vi "Find_Unmoving_Dots_in_(X,Y)-6.vi"(4 "error IN":errorcluster, 5 "Gaps for closing":i32, 6 "dR min":dbl, 7 "[IN] Primary (X,Y)":dbl[][](array[numeric])) -> (0 "error OUT":errorcluster, 1 "[OUT] Stationary Dots":T1(array[cluster]), 2 "[OUT] Dot matrix\nwith statuses for\nmoving and poten-\ntially moving dots":i16[][](array[numeric]), 3 "[OUT] (X,Y) Potentially Moving":dbl[][](array[numeric]))   [LabVIEW 2013]
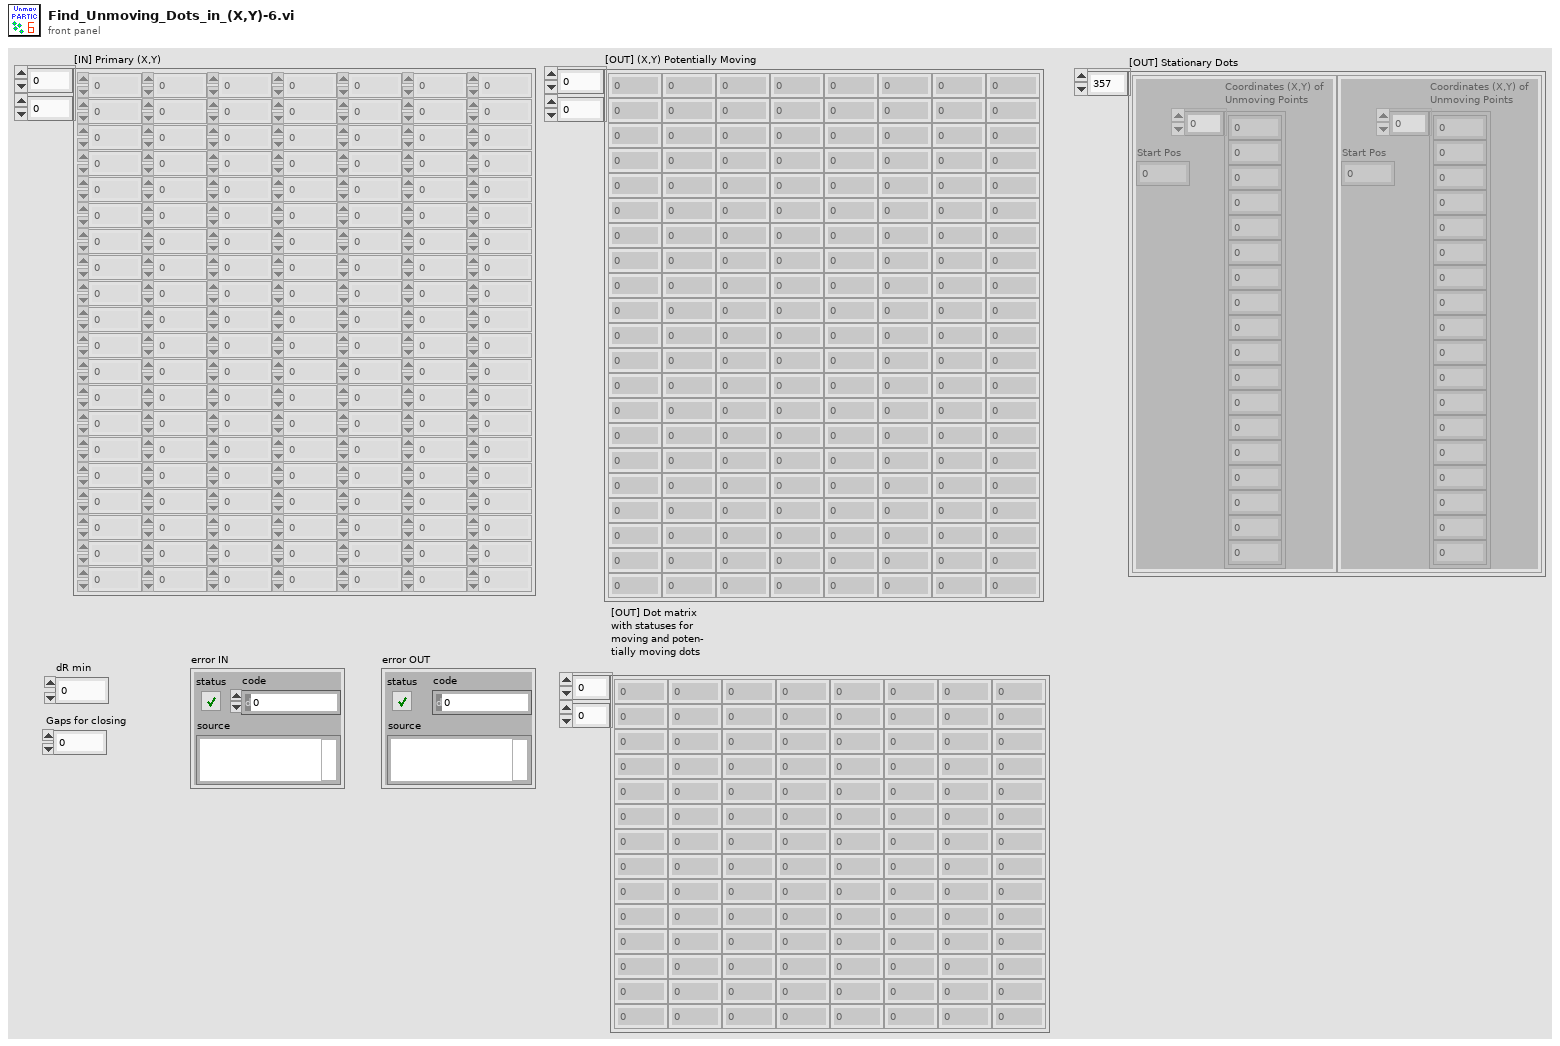
[diagram p1: front panel]
types:
  T1 = cluster{"Coordinates (X,Y) of\nUnmoving Points":dbl[], "Start Pos":i32}[]
  T2 = cluster{"Coordinates (X,Y) of\nUnmoving Points":dbl[], "Start Pos":i32}
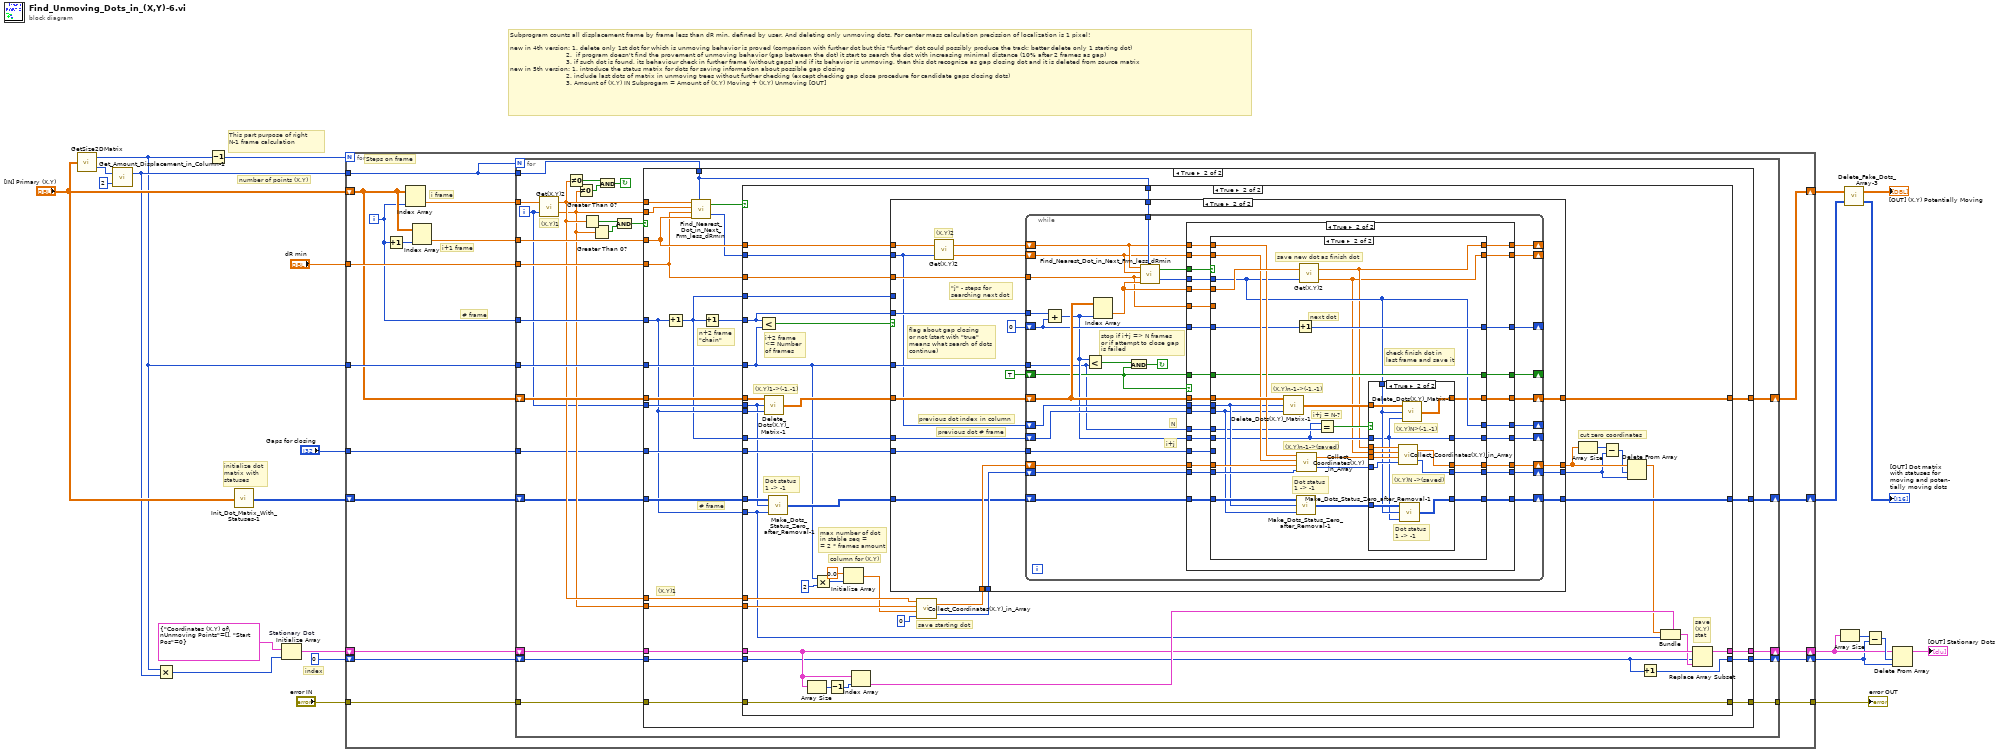
[diagram p0: block diagram]
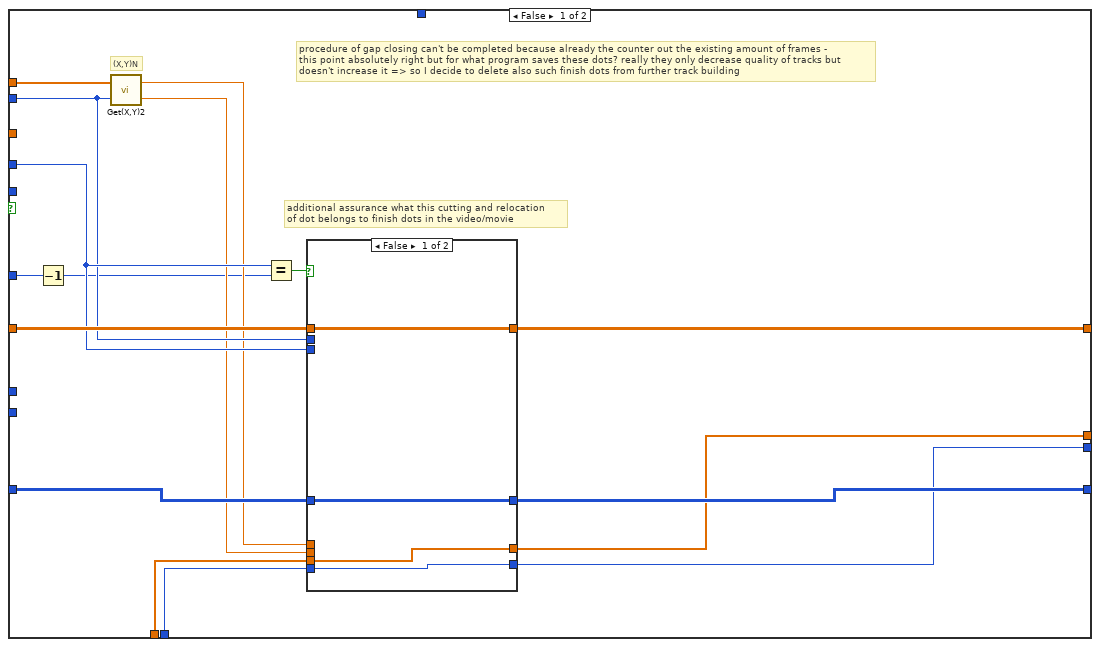
[diagram p4: hidden frame]
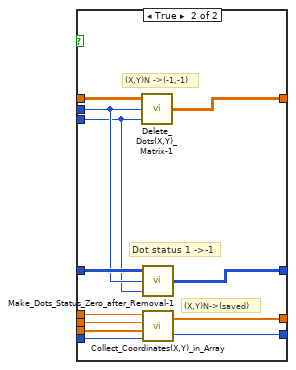
[diagram p5: hidden frame]
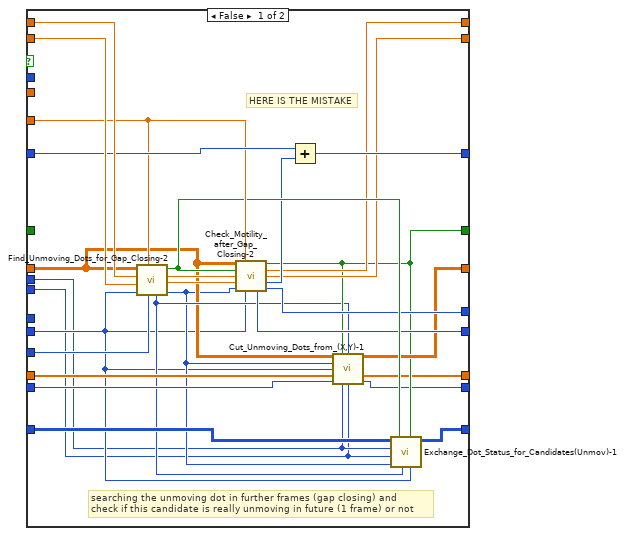
[diagram p7: hidden frame]
diagram:
  # "This part purpose of right\nN-1 frame calculation"
  # "number of points (X,Y)"
  # "initialize dot \nmatrix with \nstatuses"
  # "index"
  # "Subprogram counts all displacement frame by frame less than dR min, defined by user. And deleting only unmoving dots. For center mass calculation precission of localization is 1 pixel!\n\nnew in 4th version: 1. delete only 1st dot for which is unmoving behavior is proved (comparison with further dot but this \"further\" dot could possibly produce the track; better delete only 1 starting dot)\n                            2.  if program doesn't find the provement of unmoving behavior (gap between the dot) it start to search the dot with increasing minimal distance (10% after 2 frames as gap)\n                            3. if such dot is found, its behaviour check in further frame (without gaps) and if its behavior is unmoving, then this dot recognize as gap closing dot and it is deleted from source matrix\nnew in 5th version: 1. introduce the status matrix for dots for saving information about possible gap closing\n                            2. include last dots of matrix in unmoving trees without further checking (except checking gap close procedure for candidate gaps closing dots)\n                            3. Amount of (X,Y) IN Subprogam = Amount of (X,Y) Moving + (X,Y) Unmoving [OUT]"
  n1 = call "GetSize2DMatrix.vi"("Array IN (2D)"="[IN] Primary (X,Y)") -> ("# Cols"=w6:i32, "# Rows"=w18:i32)
  n2 = call "Get_Amount_Displacement_in_Column-1.vi"("multiplier"=2 ("y"), "# Rows"=w18) -> ("Displ amount"=w10:i32)  [unwired: 1 out]
  n3 = Multiply(x=w6, y=w10) -> (x*y=w8:i32)
  n4 = Decrement(x=w6) -> (x-1=w11:i32)
  n5 = call "Init_Dot_Matrix_With_Statuses-1.vi"("[IN] Initial (X,Y) matrix"="[IN] Primary (X,Y)") -> ("[OUT] Dot matrix\nwith initial status"=w17:i16[][])
  n6 = Initialize Array "Stationary Dot"(T2 {"Coordinates (X,Y) of\nUnmoving Points"=[], "Start Pos"=0} ("element"), w8) -> (w7:T1)
  n7 = for {
    N: w11 -> [_]
    tunnel: "dR min" -> [w40]
    tunnel: w6 -> [w38]
    shift-right: [w34] -> w2
    shift-left: 0 -> [w35]
    tunnel: "Gaps for closing" -> [w30]
    tunnel: "error IN" -> [w33]
    tunnel: [w32] -> w20
    shift-right: [w29] -> w16
    shift-left: "[IN] Primary (X,Y)" -> [w37]
    tunnel: w10 -> [w31]
    shift-right: [w27] -> w15
    shift-left: w17 -> [w28]
    shift-right: [w25] -> w3
    shift-left: w7 -> [w26]
    i -> [w36]
    # "# frame"
    # "Steps on frame"
    # "i+1 frame"
    # "i frame"
    n8 = Increment(x=w36) -> (x+1=w39:i32)
    n9 = Index Array(array=w37, index (col)=w36) -> (element=w42:dbl[])  [unwired: 1 in]
    n10 = Index Array(array=w37, index (col)=w39) -> (element=w41:dbl[])  [unwired: 1 in]
    n11 = for {
      N: w31 -> [_]
      tunnel: w42 -> [w68]
      tunnel: w41 -> [w64]
      tunnel: w31 -> [w63]
      tunnel: w40 -> [w58]
      tunnel: w38 -> [w62]
      tunnel: w36 -> [w60]
      shift-right: [w57] -> w34
      shift-left: w35 -> [w59]
      tunnel: w33 -> [w56]
      tunnel: [w55] -> w32
      shift-right: [w54] -> w29
      shift-left: w37 -> [w61]
      tunnel: w30 -> [w47]
      shift-right: [w45] -> w27
      shift-left: w28 -> [w46]
      shift-right: [w43] -> w25
      shift-left: w26 -> [w44]
      i -> [w48]
      stop <- w65 continue-if-true
      # "(X,Y)1"
      n12 = call "Get(X,Y)2.vi"("[IN] index of (X,Y)"=w48, "[IN] Array coordi\nnates (X,Y) in Frame"=w68) -> ("[OUT] Y"=w52:dbl, "[OUT] X"=w53:dbl)
      n13 = Not Equal To 0?(x=w53) -> (x != 0?=w66:bool)
      n14 = Not Equal To 0?(x=w52) -> (x != 0?=w67:bool)
      n15 = Greater Than 0?(x=w53) -> (x > 0?=w51:bool)
      n16 = Greater Than 0?(x=w52) -> (x > 0?=w50:bool)
      n17 = And(x=w66, y=w67) -> (x .and. y?=w65:bool)
      n18 = And(x=w51, y=w50) -> (x .and. y?=w49:bool)
      n19 = case shown="True" w49 {
        tunnel: w53 -> [_ w87]
        tunnel: w52 -> [_ w86]
        tunnel: w64 -> [_ w85]
        tunnel: w63 -> [_ w84]
        tunnel: w58 -> [_ w81]
        tunnel: w62 -> [_ w98]
        tunnel: w61 -> [w71 w93]
        tunnel: w60 -> [_ w78]
        tunnel: w59 -> [w73 w97]
        tunnel: w52 -> [_ w96]
        tunnel: w53 -> [_ w95]
        tunnel: [w73 w94] -> w57
        tunnel: w56 -> [w72 w92]
        tunnel: [w72 w91] -> w55
        tunnel: [w71 w90] -> w54
        tunnel: w48 -> [_ w88]
        tunnel: w47 -> [_ w80]
        tunnel: w46 -> [w70 w79]
        tunnel: [w70 w77] -> w45
        tunnel: w44 -> [w69 w75]
        tunnel: [w69 w74] -> w43
        frame False {
        }
        frame True {
          # "# frame"
          # "(X,Y)1"
          # "n+2 frame \n\"chain\""
          n20 = Increment(x=w78) -> (x+1=w76:i32)
          n21 = call "Find_Nearest_Dot_in_Next_Frm_less_dRmin.vi"("X"=w87, "Y"=w86, "dR min"=w81, "n+1 frame\ncolumn (X,Y)"=w85, "Max number\nof dots in \ncolumn (X,Y)"=w84) -> ("Any dots found?"=w82:bool, "index of the dot \nwith minimal displ"=w83:i32)
          n22 = Increment(x=w76) -> (x+1=w89:i32)
          n23 = case shown="True" w82 {
            tunnel: w98 -> [_ w119]
            tunnel: w83 -> [_ w138]
            tunnel: w97 -> [w103 w110]
            tunnel: w96 -> [_ w132]
            tunnel: w95 -> [_ w133]
            tunnel: w89 -> [_ w144]
            tunnel: w85 -> [_ w143]
            tunnel: w81 -> [_ w142]
            tunnel: [w103 w109] -> w94
            tunnel: w93 -> [w101 w139]
            tunnel: w92 -> [w102 w141]
            tunnel: [w102 w141] -> w91
            tunnel: w84 -> [_ w140]
            tunnel: [w101 w137] -> w90
            tunnel: w88 -> [_ w126]
            tunnel: w78 -> [_ w136]
            tunnel: w76 -> [_ w129]
            tunnel: w80 -> [_ w128]
            tunnel: w79 -> [w100 w127]
            tunnel: w78 -> [_ w114]
            tunnel: [w100 w124] -> w77
            tunnel: w76 -> [_ w123]
            tunnel: w75 -> [w99 w113]
            tunnel: [w99 w111] -> w74
            frame False {
            }
            frame True {
              # "save\n(X,Y)\nstat"
              # "cut zero coordinates"
              # "column for (X,Y)"
              # "max number of dot \nin stable seq = \n= 2 * frames amount"
              # "Dot status\n1 -> -1"
              # "(X,Y)1->(-1,-1)"
              # "i+2 frame\n<= Number \nof frames"
              # "save starting dot"
              n24 = Less?(x=w144, y=w119) -> (x < y?=w145:bool)
              n25 = call "Delete_Dots(X,Y)_Matrix-1.vi"("# Frame"=w136, "# Dot"=w126, "(X,Y) IN"=w139) -> ("(X,Y) OUT"=w135:dbl[][])
              n26 = call "Make_Dots_Status_Zero_after_Removal-1.vi"("# Frame"=w114, "# Dot"=w126, "[IN] Dot matrix\nwith initial status"=w127) -> ("[IN] Dot matrix\nwith zero deleted\ndots"=w125:i16[][])
              n27 = Array Size(array=w113) -> (size(s)=w117:i32)
              n28 = Multiply(x=w119, y=2) -> (x*y=w122:i32)
              n29 = Decrement(x=w117) -> (x-1=w116:i32)
              n30 = Initialize Array(0.0 ("element"), w122) -> (w118:dbl[])
              n31 = Index Array(array=w113, index=w116) -> (element=w115:T2)
              n32 = call "Collect_Coordinates(X,Y)_in_Array.vi"("Initial Index \nfor Replacement"=0, "[IN] Array for \nCollecting \nCoord (X,Y)"=w118, "Y"=w132, "X"=w133) -> ("Finish\nIndex"=w130:i32, "[OUT] Array\nfor collecting"=w131:dbl[])
              n33 = case shown="True" w145 {
                tunnel: w119 -> [w148 w197]
                tunnel: w144 -> [_ w196]
                tunnel: w138 -> [w152 w182]
                tunnel: w143 -> [w153 w194]
                tunnel: w142 -> [_ w192]
                tunnel: [w149 w189] -> w107
                tunnel: w140 -> [_ w188]
                tunnel: [w158 w187] -> w137
                tunnel: w135 -> [w161 w184]
                tunnel: w131 -> [w155 w186]
                tunnel: w130 -> [w154 w185]
                tunnel: w129 -> [_ w183]
                tunnel: w128 -> [_ w181]
                tunnel: w125 -> [w157 w180]
                tunnel: [w156 w179] -> w124
                tunnel: w123 -> [w159 _]
                tunnel: [w146 w178] -> w106
                frame False {
                  # "(X,Y)N"
                  # "additional assurance what this cutting and relocation \nof dot belongs to finish dots in the video/movie"
                  # "procedure of gap closing can't be completed because already the counter out the existing amount of frames - \nthis point absolutely right but for what program saves these dots? really they only decrease quality of tracks but\ndoesn't increase it => so I decide to delete also such finish dots from further track building"
                  n34 = Decrement(x=w148) -> (x-1=w147:i32)
                  n35 = call "Get(X,Y)2.vi"("[IN] index of (X,Y)"=w152, "[IN] Array coordi\nnates (X,Y) in Frame"=w153) -> ("[OUT] Y"=w151:dbl, "[OUT] X"=w150:dbl)
                  n36 = Equal?(x=w159, y=w147) -> (x = y?=w160:bool)
                  n37 = case shown="False" w160 {
                    tunnel: w161 -> [w165 w177]
                    tunnel: w159 -> [_ w173]
                    tunnel: w152 -> [_ w174]
                    tunnel: [w165 w176] -> w158
                    tunnel: w157 -> [w164 w175]
                    tunnel: [w164 w172] -> w156
                    tunnel: w155 -> [w163 w171]
                    tunnel: w154 -> [w162 w170]
                    tunnel: w151 -> [_ w169]
                    tunnel: w150 -> [_ w168]
                    tunnel: [w163 w167] -> w149
                    tunnel: [w162 w166] -> w146
                    frame False {
                    }
                    frame True {
                      # "(X,Y)N->(saved)"
                      # "Dot status 1 ->-1"
                      # "(X,Y)N ->(-1,-1)"
                      n38 = call "Delete_Dots(X,Y)_Matrix-1.vi"("# Frame"=w173, "# Dot"=w174, "(X,Y) IN"=w177) -> ("(X,Y) OUT"=w176:dbl[][])
                      n39 = call "Make_Dots_Status_Zero_after_Removal-1.vi"("# Frame"=w173, "# Dot"=w174, "[IN] Dot matrix\nwith initial status"=w175) -> ("[IN] Dot matrix\nwith zero deleted\ndots"=w172:i16[][])
                      n40 = call "Collect_Coordinates(X,Y)_in_Array.vi"("Initial Index \nfor Replacement"=w170, "[IN] Array for \nCollecting \nCoord (X,Y)"=w171, "Y"=w169, "X"=w168) -> ("Finish\nIndex"=w166:i32, "[OUT] Array\nfor collecting"=w167:dbl[])
                    }
                  }
                }
                frame True {
                  # "flag about gap closing\nor not (start with \"true\"\nmeans what search of dots\ncontinue)"
                  # "previous dot index in column"
                  # "previous dot # frame"
                  # "(X,Y)2"
                  # "\"j\" - steps for\nsearching next dot"
                  n41 = call "Get(X,Y)2.vi"("[IN] index of (X,Y)"=w182, "[IN] Array coordi\nnates (X,Y) in Frame"=w194) -> ("[OUT] Y"=w193:dbl, "[OUT] X"=w195:dbl)
                  n42 = while {
                    tunnel: w197 -> [w198]
                    tunnel: w196 -> [w228]
                    shift-right: [w227] -> _
                    shift-left: w195 -> [w220]
                    shift-right: [w226] -> _
                    shift-left: w193 -> [w219]
                    tunnel: w192 -> [w202]
                    shift-right: [w212] -> w189
                    shift-left: w186 -> [w215]
                    shift-right: [w213] -> w178
                    shift-left: w185 -> [w214]
                    shift-right: [w208] -> _
                    shift-left: 0 -> [w209]
                    shift-right: [w207] -> _
                    shift-left: TRUE -> [w201]
                    tunnel: w188 -> [w221]
                    shift-right: [w223] -> w187
                    shift-left: w184 -> [w222]
                    shift-right: [w204] -> _
                    shift-left: w183 -> [w210]
                    shift-right: [w206] -> _
                    shift-left: w182 -> [w211]
                    tunnel: w181 -> [w203]
                    shift-right: [w199] -> w179
                    shift-left: w180 -> [w200]
                    stop <- w224 continue-if-true
                    # "i+j"
                    # "N"
                    # "stop if i+j => N frames \nor if attempt to close gap \nis failed"
                    n43 = Add(x=w228, y=w209) -> (x+y=w205:i32)
                    n44 = Less?(x=w205, y=w198) -> (x < y?=w225:bool)
                    n45 = Index Array(array=w222, index (col)=w205) -> (element=w216:dbl[])  [unwired: 1 in]
                    n46 = And(x=w225, y=w201) -> (x .and. y?=w224:bool)
                    n47 = call "Find_Nearest_Dot_in_Next_Frm_less_dRmin.vi"("X"=w220, "Y"=w219, "dR min"=w202, "n+1 frame\ncolumn (X,Y)"=w216, "Max number\nof dots in \ncolumn (X,Y)"=w221) -> ("Any dots found?"=w217:bool, "index of the dot \nwith minimal displ"=w218:i32)
                    n48 = case shown="True" w201 {
                      tunnel: [w235 w265] -> w227
                      tunnel: [w234 w264] -> w226
                      tunnel: [w238 w263] -> w223
                      tunnel: w222 -> [w238 w262]
                      tunnel: w220 -> [w235 w261]
                      tunnel: w219 -> [w234 w260]
                      tunnel: w218 -> [_ w259]
                      tunnel: w217 -> [_ w258]
                      tunnel: w216 -> [_ w257]
                      tunnel: w215 -> [w231 w256]
                      tunnel: w214 -> [w230 w255]
                      tunnel: [w230 w254] -> w213
                      tunnel: [w231 w253] -> w212
                      tunnel: w211 -> [w233 w252]
                      tunnel: w210 -> [w232 w251]
                      tunnel: w209 -> [w236 w250]
                      tunnel: [w236 w249] -> w208
                      tunnel: w201 -> [w237 w248]
                      tunnel: [w237 w247] -> w207
                      tunnel: [w233 w246] -> w206
                      tunnel: w205 -> [_ w245]
                      tunnel: [w232 w244] -> w204
                      tunnel: w203 -> [_ w243]
                      tunnel: w202 -> [_ w242]
                      tunnel: w200 -> [w229 w241]
                      tunnel: [w229 w240] -> w199
                      tunnel: w198 -> [_ w239]
                      frame False {
                        # "gap closing procedure failed! \nSo, all data just are transfered through cycle"
                      }
                      frame True {
                        n49 = case shown="True" w258 {
                          tunnel: [w281 w297] -> w265
                          tunnel: [w280 w296] -> w264
                          tunnel: w262 -> [w272 w320]
                          tunnel: w261 -> [w293 w318]
                          tunnel: w260 -> [w292 w317]
                          tunnel: [w275 w302] -> w263
                          tunnel: w259 -> [_ w303]
                          tunnel: w257 -> [_ w319]
                          tunnel: w256 -> [w277 w316]
                          tunnel: w255 -> [w276 w315]
                          tunnel: [w268 w298] -> w254
                          tunnel: [w269 w300] -> w253
                          tunnel: w252 -> [w267 w310]
                          tunnel: w251 -> [w266 w309]
                          tunnel: w250 -> [w290 w314]
                          tunnel: [w289 w313] -> w249
                          tunnel: w248 -> [_ w312]
                          tunnel: [w274 w312] -> w247
                          tunnel: [w278 w303] -> w246
                          tunnel: w245 -> [w270 w306]
                          tunnel: [w279 w308] -> w244
                          tunnel: w243 -> [w291 _]
                          tunnel: w242 -> [w286 _]
                          tunnel: w241 -> [w288 w311]
                          tunnel: [w287 w294] -> w240
                          tunnel: w239 -> [_ w307]
                          frame False {
                            # "HERE IS THE MISTAKE"
                            # "searching the unmoving dot in further frames (gap closing) and \ncheck if this candidate is really unmoving in future (1 frame) or not"
                            n50 = call "Find_Unmoving_Dots_for_Gap_Closing-2.vi"("Gaps for closing"=w291, "dR min"=w286, "i+j"=w270, "Y"=w292, "X"=w293, "(X,Y) IN"=w272) -> ("Count of \ngaps between\ndots"=w271:i32, "Y OUT"=w283:dbl, "X OUT"=w284:dbl, "Gap Potentially \nClosed"=w285:bool, "Index of \ncandidate dot\ninside the frame"=w273:i32)  [unwired: 1 in]
                            n51 = call "Check_Motility_after_Gap_Closing-2.vi"("(X,Y) IN"=w272, "dR min"=w286, "??? Gap closed potentially ???"=w285, "X"=w284, "Y"=w283, "Count of \ngaps between\ndots"=w271, "i+j (index\nof dot before\ngap closing)"=w270) -> ("Gap closed!!!"=w274:bool, "X OUT"=w281:dbl, "Y OUT"=w280:dbl, "[OUT] Count \nof gapes + \nnext dot in \nsearching"=w282:i32, "[OUT] current dot\n# frame (column)"=w279:i32, "[OUT] current # dot\nin the frame (column)"=w278:i32)  [unwired: 3 in]
                            n52 = Add(x=w290, y=w282) -> (x+y=w289:i32)
                            n53 = call "Cut_Unmoving_Dots_from_(X,Y)-1.vi"("[IN] (X,Y)"=w272, "Gap closed!!!"=w274, "Index of \ncandidate dot\ninside the frame"=w273, "Count of gaps \nbetween dots"=w271, "i+j"=w270, "[IN] Array for collecting \nunmoving dots tree"=w277, "Starting\nIndex for\nUnmov Tree"=w276, "previous dot\nindex in column"=w267, "previous \ndot # frame"=w266) -> ("[OUT] (X,Y)"=w275:dbl[][], "[OUT] Array for collecting \nunmoving dots tree"=w269:dbl[], "Finish\nIndex"=w268:i32)  [unwired: 4 in]
                            n54 = call "Exchange_Dot_Status_for_Candidates(Unmov)-1.vi"("i+j"=w270, "Gap closed!!!"=w274, "Index of \ncandidate dot\ninside the frame"=w273, "Gap Potentially \nClosed"=w285, "Count of potentially\ngaps between dots"=w271, "previous dot\n# frame"=w266, "previous dot\nindex in column"=w267, "[IN] Dot matrix with zero \ndeleted dots"=w288) -> ("[OUT] Dot matrix with zero \ndeleted dots"=w287:i16[][])  [unwired: 3 in]
                          }
                          frame True {
                            # "check finish dot in\nlast frame and save it"
                            # "i+j = N-?"
                            # "Dot status\n1 -> -1"
                            # "(X,Y)n-1->(saved)"
                            # "next dot"
                            # "save new dot as finish dot"
                            # "(X,Y)n-1->(-1,-1)"
                            n55 = call "Delete_Dots(X,Y)_Matrix-1.vi"("# Frame"=w309, "# Dot"=w310, "(X,Y) IN"=w320) -> ("(X,Y) OUT"=w304:dbl[][])
                            n56 = Increment(x=w314) -> (x+1=w313:i32)
                            n57 = call "Make_Dots_Status_Zero_after_Removal-1.vi"("# Frame"=w309, "# Dot"=w310, "[IN] Dot matrix\nwith initial status"=w311) -> ("[IN] Dot matrix\nwith zero deleted\ndots"=w295:i16[][])
                            n58 = call "Collect_Coordinates(X,Y)_in_Array.vi"("Initial Index \nfor Replacement"=w315, "[IN] Array for \nCollecting \nCoord (X,Y)"=w316, "Y"=w317, "X"=w318) -> ("Finish\nIndex"=w299:i32, "[OUT] Array\nfor collecting"=w301:dbl[])
                            n59 = call "Get(X,Y)2.vi"("[IN] index of (X,Y)"=w303, "[IN] Array coordi\nnates (X,Y) in Frame"=w319) -> ("[OUT] Y"=w296:dbl, "[OUT] X"=w297:dbl)
                            n60 = Equal?(x=w306, y=w307) -> (x = y?=w305:bool)
                            n61 = case shown="True" w305 {
                              tunnel: w306 -> [w325 w326]
                              tunnel: [w325 w326] -> w308
                              tunnel: w304 -> [w324 w337]
                              tunnel: w303 -> [_ w327]
                              tunnel: [w324 w336] -> w302
                              tunnel: w301 -> [w323 w335]
                              tunnel: [w323 w332] -> w300
                              tunnel: w299 -> [w322 w334]
                              tunnel: [w322 w333] -> w298
                              tunnel: w297 -> [_ w331]
                              tunnel: w296 -> [_ w330]
                              tunnel: w295 -> [w321 w329]
                              tunnel: [w321 w328] -> w294
                              frame False {
                              }
                              frame True {
                                # "Dot status\n1 -> -1"
                                # "(X,Y)N ->(saved)"
                                # "(X,Y)N>(-1,-1)"
                                n62 = call "Collect_Coordinates(X,Y)_in_Array.vi"("Initial Index \nfor Replacement"=w334, "[IN] Array for \nCollecting \nCoord (X,Y)"=w335, "Y"=w330, "X"=w331) -> ("Finish\nIndex"=w333:i32, "[OUT] Array\nfor collecting"=w332:dbl[])
                                n63 = call "Make_Dots_Status_Zero_after_Removal-1.vi"("# Frame"=w326, "# Dot"=w327, "[IN] Dot matrix\nwith initial status"=w329) -> ("[IN] Dot matrix\nwith zero deleted\ndots"=w328:i16[][])
                                n64 = call "Delete_Dots(X,Y)_Matrix-1.vi"("# Frame"=w326, "# Dot"=w327, "(X,Y) IN"=w337) -> ("(X,Y) OUT"=w336:dbl[][])
                              }
                            }
                          }
                        }
                      }
                    }
                  }
                }
              }
              n65 = Array Size(array=w107) -> (size(s)=w108:i32)
              n66 = Subtract(x=w108, y=w106) -> (x-y=w105:i32)
              n67 = Delete From Array(array=w107, length=w105, index=w106) -> (array with subset deleted=w104:dbl[])  [unwired: 1 out]
              n68 = Increment(x=w110) -> (x+1=w109:i32)
              n69 = Bundle(cluster=w115, "Coordinates (X,Y) of\nUnmoving Points"=w104, "Start Pos"=w114) -> (w112:T2)
              n70 = Replace Array Subset(array=w113, new element=w112, index=w110) -> (w111:T1)
            }
          }
        }
      }
    }
  }
  "error OUT" <- w20
  n71 = Array Size(array=w3) -> (size(s)=w5:i32)
  n72 = call "Delete_Fake_Dots_Array-3.vi"("[IN] Dot matrix\nwith initial status"=w15, "[IN] Source \nArray"=w16) -> ("[OUT] Dot \nMatrix"=→"[OUT] Dot matrix\nwith statuses for\nmoving and poten-\ntially moving dots":i16[][], "[OUT] Filtered \nArray (X,Y)"=→"[OUT] (X,Y) Potentially Moving":dbl[][])
  n73 = Subtract(x=w5, y=w2) -> (x-y=w4:i32)
  n74 = Delete From Array(array=w3, length=w4, index=w2) -> (array with subset deleted=→"[OUT] Stationary Dots":T1)  [unwired: 1 out]
